vi "Get Object Attributes.vi"(8 "error in (no error)":errorcluster, 10 "Object ID":i32=-1, 11 "Attributes in":refnum<class "Attributes.lvclass">) -> (0 "error out":errorcluster, 1 "Attributes":refnum<class "Attribute.lvclass">[](array[class]), 3 "Attributes out":refnum<class "Attributes.lvclass">)   [LabVIEW 2019, in "HierDAL Library.lvlib" / "Database.lvlib" / "Repositories.lvlib" / "Attributes.lvclass"]
uses:
  Attributes.lvclass
  Models Library/Attribute Class/Attribute.lvclass
  Attributes.lvclass/Attributes.ctl
  Database Manager Class/Database Manager.lvclass
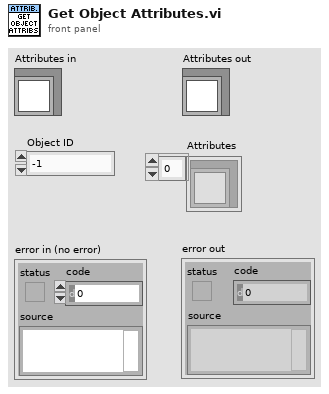
[diagram p1: front panel]
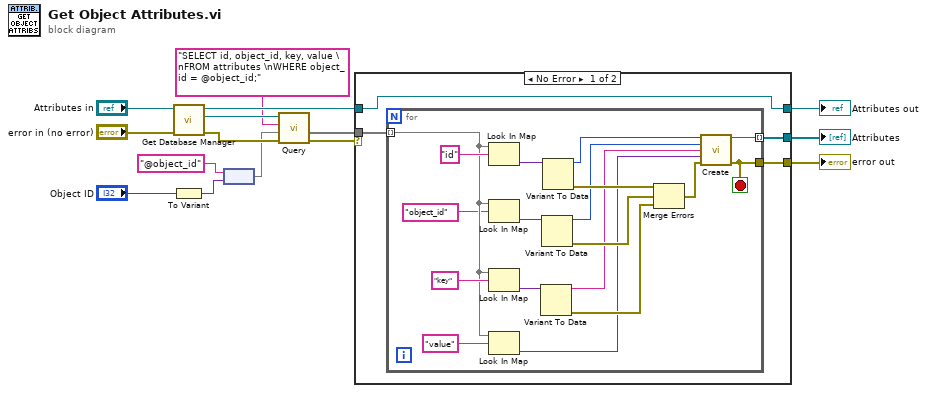
[diagram p0: block diagram]
diagram:
  n1 = call "Get Database Manager.vi"("error in (no error)"="error in (no error)", "Attributes in"="Attributes in") -> ("error out"=w14:errorcluster, "Database Manager"=w13:refnum<class "Database Manager.lvclass">, "Attributes out"=w15:refnum<class "Attributes.lvclass">)  [unwired: 7 in]
  n2 = To Variant(anything="Object ID") -> (Variant=w4:variant)
  n3 = node("@object_id" ("key"), w4) -> (w2:map{string, variant})
  n4 = call-dynamic "Query.vi"("error in (no error)"=w14, "Parameters"=w2, "Query"="SELECT id, object_id, key, value \nFROM attributes \nWHERE object_id = @object_id;", "Database Manager in"=w13) -> ("error out"=w7:errorcluster, "Rows"=w9:map{string, variant}[])  [unwired: 5 in, 1 out]
  n5 = case shown="No Error" w7 {
    selector: w7 -> [_ w38]
    tunnel: [w19 _] -> w5
    tunnel: w9 -> [w16 _]
    tunnel: [w18 w38] -> w8
    tunnel: w15 -> [w17 w39]
    tunnel: [w17 w39] -> w6
    frame No Error {
      n6 = for {
        tunnel: [w23] -> w19 mode=indexing
        tunnel: [w22] -> w18
        tunnel: w16 -> [w21] mode=indexing
        stop <- w22 stop-if-true
        n7 = Look In Map(map=w21, key="id") -> (value=w36:variant)  [unwired: 1 in, 1 out]
        n8 = Look In Map(map=w21, key="object_id") -> (value=w35:variant)  [unwired: 1 in, 1 out]
        n9 = Look In Map(map=w21, key="key") -> (value=w29:variant)  [unwired: 1 in, 1 out]
        n10 = Look In Map(map=w21, key="value") -> (value=w26:variant)  [unwired: 1 in, 1 out]
        n11 = Variant To Data(Variant=w29) -> (data=w27:string, error out=w28:errorcluster)  [unwired: 2 in]
        n12 = Variant To Data(Variant=w35) -> (data=w31:i32, error out=w33:errorcluster)  [unwired: 2 in]
        n13 = Variant To Data(Variant=w36) -> (data=w32:i32, error out=w34:errorcluster)  [unwired: 2 in]
        n14 = Merge Errors(w34, w33, w28) -> (w30:errorcluster)
        n15 = call "Create.vi"("ID"=w32, "Object ID"=w31, "Key"=w27, "Value"=w26, "error in (no error)"=w30) -> ("Attribute out"=w23:refnum<class "Attribute.lvclass">, "error out"=w22:errorcluster)  [unwired: 9 in]
      }
    }
    frame Error {
    }
  }
  "error out" <- w8
  "Attributes out" <- w6
  "Attributes" <- w5
